vi "Measurement_input_panel.vi"(0 "OK":T4, 2 "setup":T5, 5 "Setup filename":string) -> (11 "Setup filename out":string, 12 "Analysis Info cluster":T8[](array[typedef])=[{"Colour"=0, "Inst type"=enum."Pitot-static tube", "Inst name"="Manometer voltage", "Symbol"="U", "Code name"="", "Extra Info"="U", "Inst Array"=enum."PWA", "Extra Titles"=[], "Extra Values"=[], "U"=0.0, "u^2"=0.0, "u^3"=0.0, "u^4"=0.0, "Skew_u"=0.0, "Kurt_u"=0.0, "Sd Error in Mean"=0.0, "% u'/U"=0.0, "X"=0.0, "Y"=0.0, "Z"=0.0, "Timescale integral to 25%"=0.0, "Sd Error in Variance"=0.0, "Calib File"=path "", "Calib Constants"=[], "Output Position"=FALSE, "Full Stats"=FALSE, "Av Sampling Rate"=0.0, "Av No of Samples"=0.0, "Total Meas Time (s)"=0.0, "ADAM Ch Name"=""}, {"Colour"=0, "Inst type"=enum."Pitot-static tube", "Inst name"="Manometer voltage", "Symbol"="U", "Code name"="", "Extra Info"="U", "Inst Array"=enum."PWA", "Extra Titles"=[], "Extra Values"=[], "U"=0.0, "u^2"=0.0, "u^3"=0.0, "u^4"=0.0, "Skew_u"=0.0, "Kurt_u"=0.0, "Sd Error in Mean"=0.0, "% u'/U"=0.0, "X"=0.0, "Y"=0.0, "Z"=0.0, "Timescale integral to 25%"=0.0, "Sd Error in Variance"=0.0, "Calib File"=path "", "Calib Constants"=[], "Output Position"=FALSE, "Full Stats"=FALSE, "Av Sampling Rate"=0.0, "Av No of Samples"=0.0, "Total Meas Time (s)"=0.0, "ADAM Ch Name"=""}, {"Colour"=0, "Inst type"=enum."Pitot-static tube", "Inst name"="Manometer voltage", "Symbol"="U", "Code name"="", "Extra Info"="U", "Inst Array"=enum."PWA", "Extra Titles"=[], "Extra Values"=[], "U"=0.0, "u^2"=0.0, "u^3"=0.0, "u^4"=0.0, "Skew_u"=0.0, "Kurt_u"=0.0, "Sd Error in Mean"=0.0, "% u'/U"=0.0, "X"=0.0, "Y"=0.0, "Z"=0.0, "Timescale integral to 25%"=0.0, "Sd Error in Variance"=0.0, "Calib File"=path "", "Calib Constants"=[], "Output Position"=FALSE, "Full Stats"=FALSE, "Av Sampling Rate"=0.0, "Av No of Samples"=0.0, "Total Meas Time (s)"=0.0, "ADAM Ch Name"=""}] {"Sd Error in Variance" format="%.2f"; "Skew_u" format="%.2f"; "% u'/U" format="%.2f"; "Sd Error in Mean" format="%.2f"; "Kurt_u" format="%.2f"; "u^4" format="%.2f"; "u^3" format="%.2f"; "U" format="%.2f"; "u^2" format="%.2f"})   [LabVIEW 2013]
uses:
  Controls/Ch_and_spans_choices.ctl
  Controls/Inst_type.ctl
  Controls/Analysis_info_cluster.ctl
  Controls/Instrument_Array.ctl
  Controls/LDA_Setup.ctl
  Controls/Setup.ctl
  Controls/ok_button.ctl
  Controls/Trigger_Mode.ctl
  Controls/PWA_Data.ctl
  File/Setup_Filetype.ctl
  Controls/Post_Process.ctl
  Controls/App_Global.ctl
  Controls/Ch_and_Spans.ctl
  Globals/Meas_global.vi
  Globals/Trav_pos_global.vi
  Globals/LDA_meas_global_1.vi
  Globals/Preference_global.vi
panel:
  in  "Acquisition Plug in":u16(ring) items=["ADAM_Server_Channels.vi", "Channels_and_Index.ctl", "DataTranslation.vi", "DT_With_Multiplexer.vi", "LDA_IP.vi", "NI-DAQmx.vi", "Simulate_kernal.vi"]
  in  "Select Duplicate Channels":bool
  in  "PWA Data":T1
  out "Inst type":T2
  in  "Edit temp and Press":bool
  out "Abs Press (mbar)":dbl=1013.0 format="%.1f"
  out "Temp (deg C)":dbl=21.0 format="%.1f"
  in  "Trigger mode":T3
  in  "Select Plug Ins":bool
  in  "Sync Delay Time (ms)":dbl=24.0 format="%.2f"
  out "XW Present?":bool
  out "Read Setup File?":bool
  out "Setup Paths":string[](array[string])
  in  "Select ADAM Channels":bool
  in  "stop":bool
  out "Notes":string
  in  "Setup filename selector":u16(ring) items=["Current_Setup.xls", "Calib_Setup.xls"]
  in  "Synchronise Analogue channels with LDA":bool
  in  "LDA set up":T6={"dimensions"=enum."2D", "Analogue Freq Multiplier"=0.1} {"Analogue Freq Multiplier" min=0.1 max=100.0 format="%_5g"}
  in  "LDA data":enum16{"No LDA data", "Take LDA data"}(ring)=enum."Take LDA data"
  in  "Cross wire":T7(ring)
  in  "No of Analogue inst":i32=1
  in  "Ch & spans choices":T10[](array[typedef]) {"D" format="%.2f"; "Ch No" min=0; "low limit" min=-10 max=10 format="%.2f"; "high limit" min=-10 max=10 format="%.2f"}
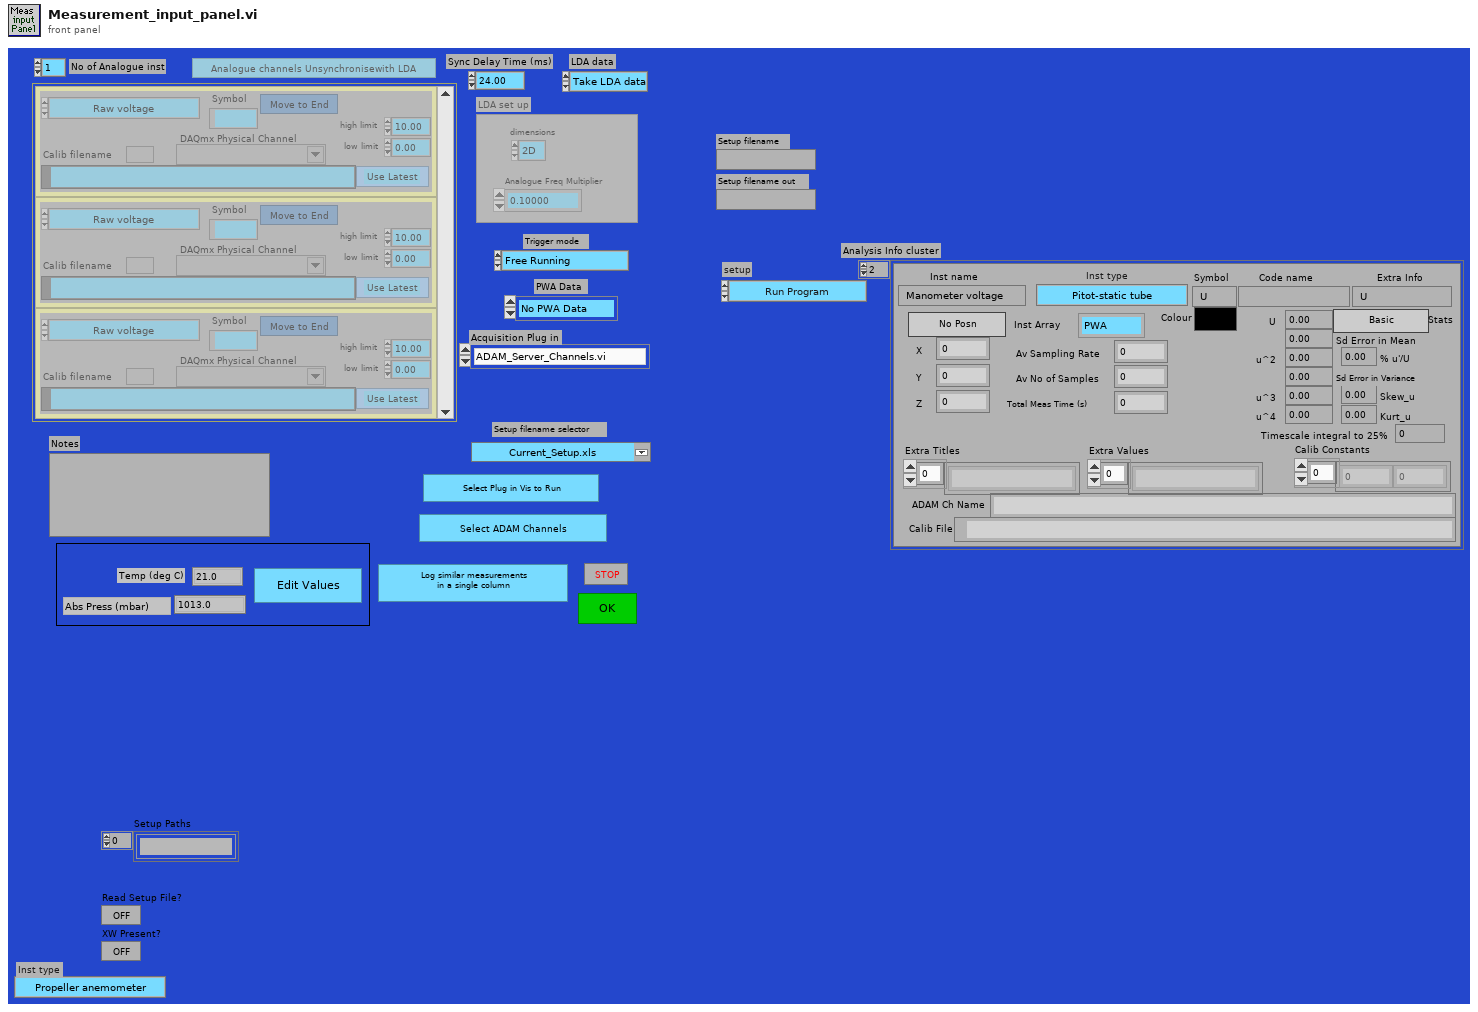
[diagram p1: front panel]
types:
  T1 = typedef "PWA_Data.ctl" = enum16{"No PWA Data", "One Ch PWA"}
  T2 = typedef "Inst_type.ctl" = enum16{"Propeller anemometer", "Raw voltage", "Pressure Transducer", "Pitot-static tube", "Preston tube", "Hot wire", "Cross wire 1", "Cross wire 2", "Generic Linear", "Generic Polynomial", "Generic BackPoly", "Fast FID", "Thermocouple", "Cold wire", "Pulsed Wire", "LDA Vel", "LDA Tran time", "LDA Arr time"}
  T3 = typedef "Trigger_Mode.ctl" = enum16{"Free Running", "Start on Trigger", "Trigger Every Block", "Trigger Every Sample"}
  T4 = typedef "ok_button.ctl" = bool
  T5 = typedef "Setup.ctl" = enum16{"Run Program", "Show Setup", "Save Current Setup", "Setup Front Panel"}
  T6 = typedef "LDA_Setup.ctl" = cluster{"dimensions":enum16{"1D", "2D"}, "Analogue Freq Multiplier":dbl}
  T7 = enum16{"2nd component as calculated", "2nd component multipled by -1"}
  T8 = typedef "Analysis_info_cluster.ctl" = cluster{"Colour":u32, "Inst type":T2, "Inst name":string, "Symbol":string, "Code name":string, "Extra Info":string, "Inst Array":T9, "Extra Titles":string[], "Extra Values":string[], "U":dbl, "u^2":dbl, "u^3":dbl, "u^4":dbl, "Skew_u":dbl, "Kurt_u":dbl, "Sd Error in Mean":dbl, "% u'/U":dbl, "X":dbl, "Y":dbl, "Z":dbl, "Timescale integral to 25%":dbl, "Sd Error in Variance":dbl, "Calib File":path, "Calib Constants":dbl[], "Output Position":bool, "Full Stats":bool, "Av Sampling Rate":dbl, "Av No of Samples":dbl, "Total Meas Time (s)":dbl, "ADAM Ch Name":string}
  T9 = typedef "Instrument_Array.ctl" = enum16{"PWA", "LDA", "Analogue"}
  T10 = typedef "Ch_and_spans_choices.ctl" = cluster{"high limit":sgl, "low limit":sgl, "Ch No":i16, "Calib filename":path, "Inst type":T2, "Symbol":string, "Move channel":bool, "Use Latest":bool, "D":dbl, "Ch Name":string, "DAQmx Physical Channel":tag}
  T11 = typedef "Post_Process.ctl" = enum16{"Take New Data", "Post Process Raw Data File"}
  T12 = typedef "Setup_Filetype.ctl" = enum16{"Measurement Setups", "Calibration Setups", "General", "Results File Plotter Setups", "Speed Calib Tweaks"}
  T13 = typedef "App_Global.ctl" = enum16{"Read Global", "Write to Global", "Initialise Array"}
  T14 = typedef "Ch_and_Spans.ctl" = cluster{"high limit (10V)":sgl, "low limit (-10V)":sgl, "Ch No":i16, "Var name":string, "Use Latest Calib":bool, "DAQmx Chan":tag}
  T15 = enum16{"Zero or one", "One", "Zero or more", "One or more"}
  T16 = typedef "Traverse_cluster.ctl" = cluster{"Start X":dbl, "Start Y":dbl, "Start Z":dbl, "End X":dbl, "End Y":dbl, "End Z":dbl, "No. of pts.":i32, "Spacing":T17, "Filename":path, "Tunnel Speed":dbl, "Averaging time (min)":dbl, "Extra Commands":string, "Specific Arguments":string, "Emission Rate (l/min)":dbl, "Trace Gas Concentration (%)":dbl, "Density Ratio":string, "Comments":string, "Row No":i32, "Row Type Selector":T18, "Completion time":string, "Row Duration (mins)":dbl, "No. of Valid pts.":i32, "Meas Setup File":string}
  T17 = typedef "Spacing.ctl" = enum16{"Linear", "Log", "Gauss", "Specified", "N/A"}
  T18 = typedef "Multi_run_mode.ctl" = enum16{"Move Traverse Only", "Set Tunnel Speed Only", "Set Source Only", "Set Measurement Conditions", "Single Measurement", "Vertical Profile", "Lateral Profile", "Longitudinal Profile", "Explore Volume", "Multi-Axis Profile", "Auto Calibrate", "Meas Fast FID Bkgnd", "Check Beam Power", "Scanning Valve Measurement", "Run VI Named:", "Set ADAM Ch", "Wait (minutes)", "Send Message", "Synchronize With:", "Fall Back to this Row", "Turn Off Row Repeating", "Blank Row", "Traverse 3D Volume"}
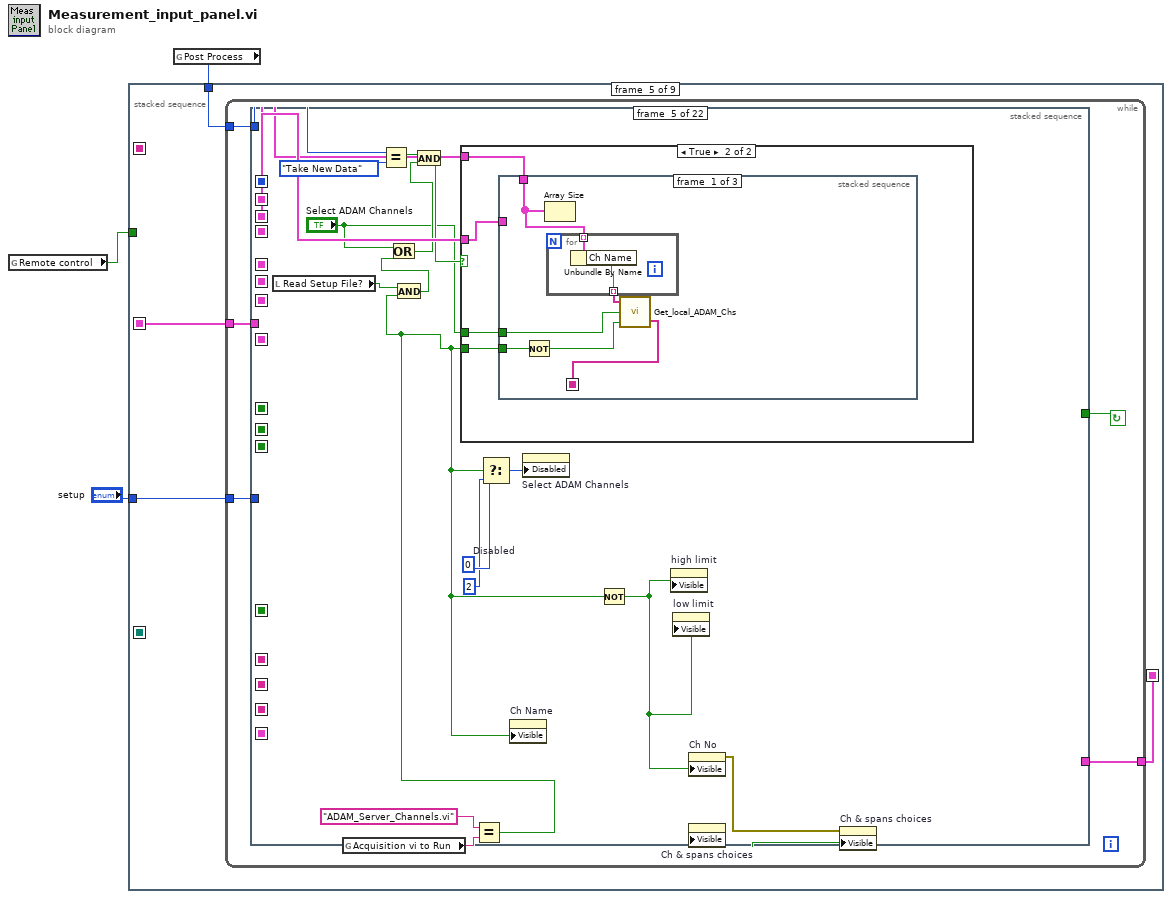
[diagram p0: block diagram]
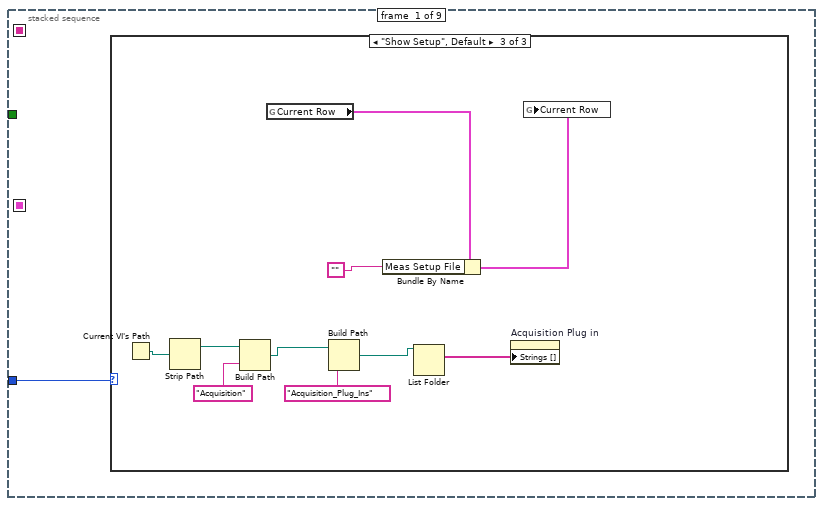
[diagram p2: hidden frame]
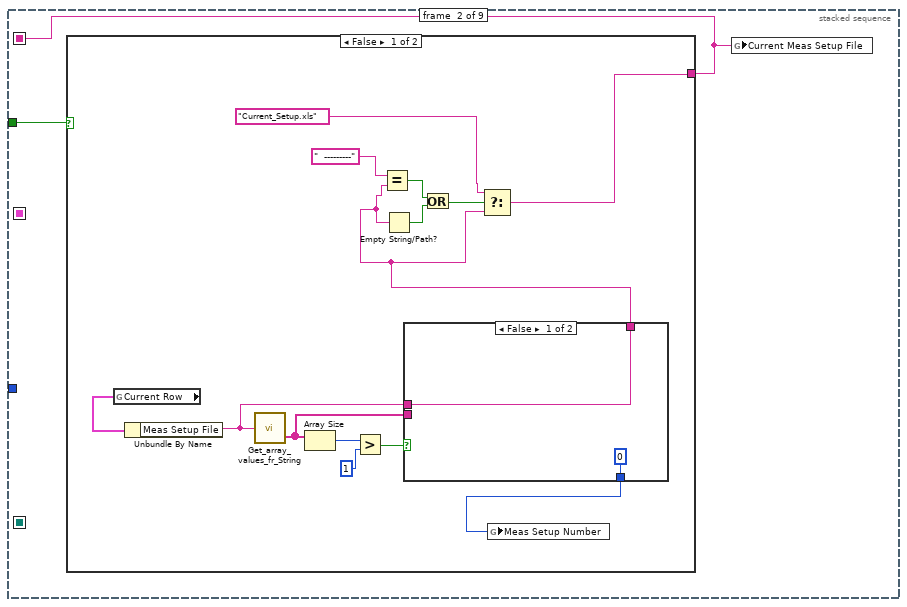
[diagram p5: hidden frame]
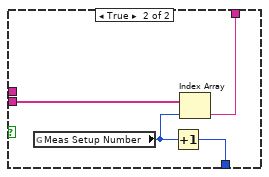
[diagram p6: hidden frame]
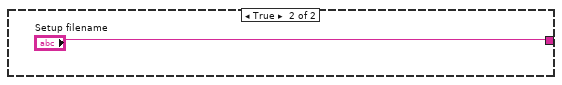
[diagram p7: hidden frame]
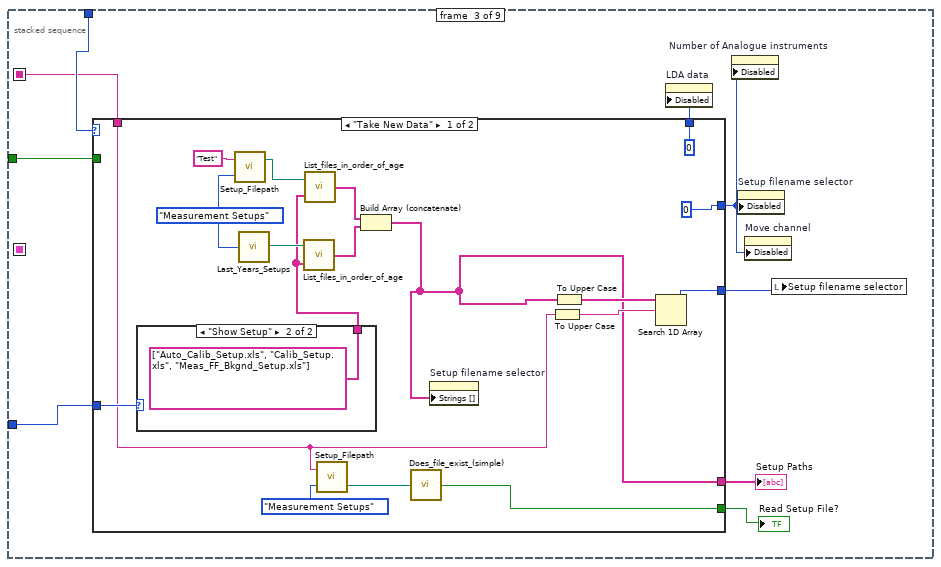
[diagram p8: hidden frame]
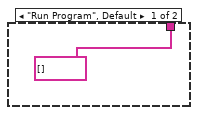
[diagram p9: hidden frame]
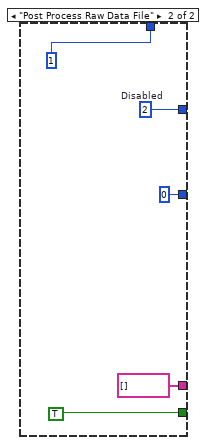
[diagram p10: hidden frame]
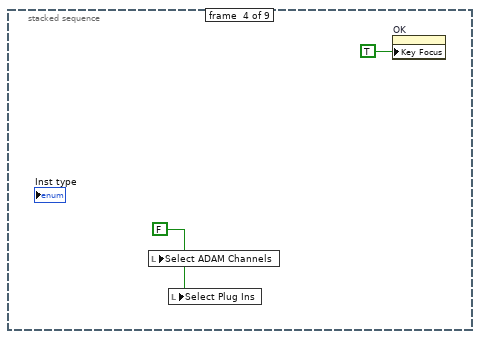
[diagram p11: hidden frame]
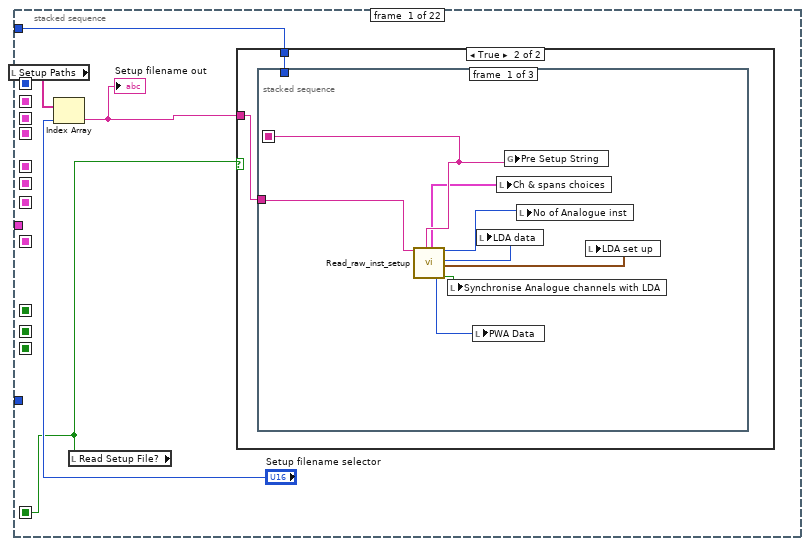
[diagram p12: hidden frame]
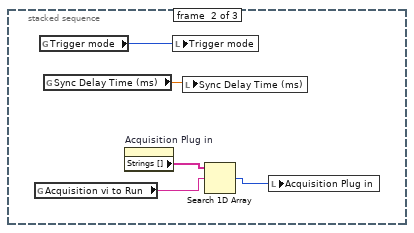
[diagram p14: hidden frame]
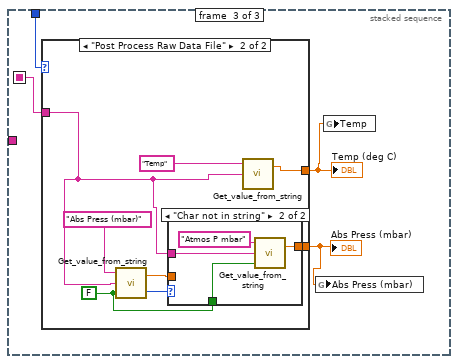
[diagram p15: hidden frame]
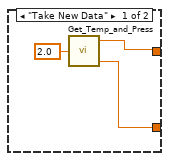
[diagram p16: hidden frame]
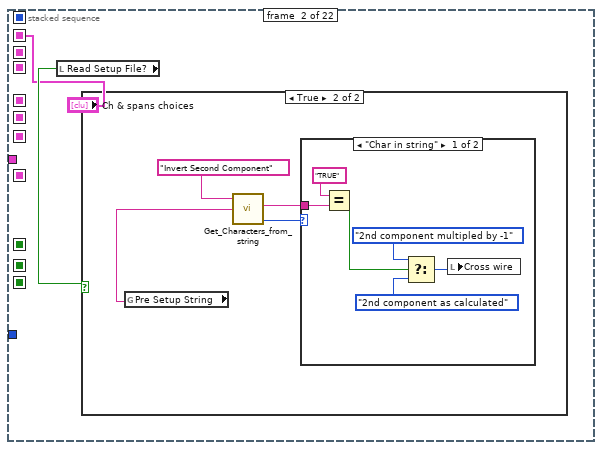
[diagram p18: hidden frame]
diagram:
  n1 = global read "Meas_global.vi" "Remote control"() -> (w1:bool)
  n2 = global read "Meas_global.vi" "Post Process"() -> (w3:T11)
  n3 = stacked-sequence {
    seq-local: [_ _ _ _ w77 _ _ _ _] -> [_ _ _ _ _ _ w748 w849 _]
    seq-local: [_ w15 _ _ _ _ _ _ _] -> [_ _ w38 _ _ _ w747 _ _]
    seq-local: [_ _ _ _ w74 _ _ _ _] -> [_ _ _ _ _ _ _ _ w912]
    seq-local: [_ _ _ _ _ _ _ w848 _] -> [_ _ _ _ _ _ _ _ w911]
    tunnel: w3 -> [_ _ w46 _ w76 _ _ w850 _]
    tunnel: "setup" -> [w4 _ w40 _ w75 _ w749 _ _]
    tunnel: w1 -> [_ w16 w39 _ _ _ _ _ _]
    frame #0 {
      n4 = case shown="\"Show Setup\", Default" w4 {
        frame "Run Program" {
        }
        frame "Setup Front Panel" {
        }
        frame "Show Setup", Default {
          n5 = Current VI's Path() -> (path=w11:path)
          n6 = Strip Path(path=w11) -> (stripped path=w10:path)  [unwired: 1 out]
          n7 = Build Path(base path=w10, name or relative path="Acquisition") -> (appended path=w7:path)
          n8 = global read "Trav_pos_global.vi" "Current Row"() -> (w14:T16)
          n9 = Build Path(base path=w7, name or relative path="Acquisition_Plug_Ins") -> (appended path=w6:path)
          n10 = Bundle By Name(cluster=w14, "Meas Setup File"="") -> (w13:T16)
          n11 = List Folder(path=w6) -> (filenames=w5:string[])  [unwired: 3 in, 3 out]
          n12 = property on="Acquisition Plug in" class="Ring (strict)"("Strings []"=w5) -> ()  [unwired: 2 in, 2 out]
          n13 = global write "Trav_pos_global.vi" "Current Row"(w13) -> ()
        }
      }
    }
    frame #1 {
      n14 = case shown="False" w16 {
        tunnel: [w29 "Setup filename"] -> w15
        frame False {
          n15 = global read "Trav_pos_global.vi" "Current Row"() -> (w25:T16)
          n16 = Unbundle By Name(w25) -> ("Meas Setup File"=w19:string)
          n17 = call "Get_array_values_fr_String.vi"("String Value"=w19) -> ("String array"=w18:string[])  [unwired: 1 out]
          n18 = Array Size(array=w18) -> (size(s)=w23:i32)
          n19 = Greater?(x=w23, y=1) -> (0:w21:bool)
          n20 = case shown="False" w21 {
            tunnel: [w32 w35] -> w20
            tunnel: w19 -> [w32 _]
            tunnel: w18 -> [_ w36]
            tunnel: [0 w33] -> w17
            frame False {
            }
            frame True {
              n21 = global read "Trav_pos_global.vi" "Meas Setup Number"() -> (w34:i32)
              n22 = Increment(x=w34) -> (x+1=w33:i32)
              n23 = Index Array(array=w36, index=w34) -> (element=w35:string)
            }
          }
          n24 = Equal?(x="  ---------" ("f"), y=w20) -> (x = y?=w28:bool)
          n25 = Empty String/Path?(string/path=w20) -> (empty?=w27:bool)
          n26 = Or(x=w28, y=w27) -> (x .or. y?=w24:bool)
          n27 = Select(t="Current_Setup.xls", s=w24, f=w20) -> (s? t:f=w29:string)
          n28 = global write "Trav_pos_global.vi" "Meas Setup Number"(w17) -> ()
        }
        frame True {
        }
      }
      n29 = global write "Trav_pos_global.vi" "Current Meas Setup File"(w15) -> ()
    }
    frame #2 {
      n30 = case shown="\"Take New Data\"" w46 {
        tunnel: [w47 string[] []] -> w42
        tunnel: [w60 TRUE ("exists")] -> w41
        tunnel: [u8 0 ("Disabled") w68] -> w43
        tunnel: [u8 0 ("Disabled") u8 1 ("Disabled")] -> w45
        tunnel: w38 -> [w56 _]
        tunnel: [w63 0 ("index of element")] -> w44
        tunnel: w40 -> [w58 _]
        tunnel: w39 -> [_ _]
        frame "Take New Data" {
          w50 = Setup_Filetype."Measurement Setups" ("Setup File Type")
          n31 = case shown="\"Show Setup\"" w58 {
            tunnel: [string[] [] ("file names") string[] ["Auto_Calib_Setup.xls", "Calib_Setup.xls", "Meas_FF_Bkgnd_Setup.xls"] ("file names")] -> w48
            frame "Run Program", Default {
            }
            frame "Show Setup" {
            }
          }
          n32 = call "Setup_Filepath.vi"("Setup File Type"=w50, "Filename in"="Test") -> ("Directory"=w51:path)  [unwired: 1 out]
          n33 = call "Last_Years_Setups.vi"("Setup File Type"=w50) -> ("Directory"=w49:path)
          n34 = call "List_files_in_order_of_age.vi"("Files to Hide"=w48, "Folder"=w49) -> ("file names"=w53:string[])
          n35 = call "List_files_in_order_of_age.vi"("Files to Hide"=w48, "Folder"=w51) -> ("file names"=w52:string[])
          n36 = call "Setup_Filepath.vi"("Setup File Type"=Setup_Filetype."Measurement Setups", "Filename in"=w56) -> ("Filename Out"=w55:path)  [unwired: 1 out]
          n37 = Build Array (concatenate)(w52, w53) -> (w47:string[])
          n38 = call "Does_file_exist_(simple).vi"("Pathname"=w55) -> ("exists?"=w60:bool)
          n39 = property on="Setup filename selector" class="Ring (strict)"("Strings []"=w47) -> ()  [unwired: 2 in, 2 out]
          n40 = To Upper Case(1:w56) -> (0:w61:string)
          n41 = To Upper Case(1:w47) -> (0:w62:string[])
          n42 = Search 1D Array(1D array=w62, element=w61) -> (index of element=w63:i32)  [unwired: 1 out]
        }
        frame "Post Process Raw Data File" {
          w68 = u8 2  # Disabled
        }
      }
      "Setup Paths" <- w42
      "Read Setup File?" <- w41
      n43 = property on="LDA data" class="Enum (strict)"("Disabled"=w45) -> ()  [unwired: 2 in, 2 out]
      n44 = property on="Number of Analogue instruments" class="DigNum (strict)"("Disabled"=w43) -> ()  [unwired: 2 in, 2 out]
      n45 = property on="Setup filename selector" class="Ring (strict)"("Disabled"=w43) -> ()  [unwired: 2 in, 2 out]
      n46 = property on="Move channel" class="Bool (strict)"("Disabled"=w43) -> ()  [unwired: 2 in, 2 out]
      n47 = local write "Setup filename selector"(w44) -> ()
    }
    frame #3 {
      w73 = FALSE ("Select Local ADAM Channels")
      n48 = local write "Select ADAM Channels"(w73) -> ()
      n49 = local write "Select Plug Ins"(w73) -> ()
      n50 = property on="OK" class="Bool"("Key Focus"=TRUE) -> ()  [unwired: 2 in, 2 out]
    }
    frame #4 {
      n51 = while {
        tunnel: w75 -> [w79]
        tunnel: w76 -> [w80]
        tunnel: [w82] -> w77
        tunnel: [w78] -> w74
        stop <- w81 continue-if-true
        n52 = stacked-sequence {
          seq-local: [_ _ _ _ _ _ _ _ _ w243 _ _ _ _ _ _ _ _ _ _ _ _] -> [_ _ _ _ _ _ _ _ _ _ _ w306 w351 w422 _ _ _ _ _ _ _ _]
          seq-local: [_ _ _ _ w166 _ _ _ _ _ _ _ _ _ _ _ _ _ _ _ _ _] -> [_ _ _ _ _ _ w205 _ w239 w244 _ _ _ _ _ _ _ _ _ _ _ _]
          seq-local: [_ _ _ _ _ _ w210 _ _ _ _ _ _ _ _ _ _ _ _ _ _ _] -> [_ _ _ _ _ _ _ _ _ w245 _ _ _ _ _ _ _ _ _ _ _ _]
          seq-local: [_ _ _ _ _ _ _ _ _ _ _ w308 _ _ _ _ _ _ _ _ _ _] -> [_ _ _ _ _ _ _ _ _ _ _ _ w353 _ _ _ _ _ _ _ _ w713]
          seq-local: [_ _ _ _ _ _ _ _ _ _ _ _ _ _ w470 _ _ _ _ _ _ _] -> [_ _ _ _ _ _ _ _ _ _ _ _ _ _ _ w495 _ _ _ _ _ _]
          seq-local: [_ _ _ _ _ _ _ _ _ _ _ _ _ _ _ w491 _ _ _ _ _ _] -> [_ _ _ _ _ _ _ _ _ _ _ _ _ _ _ _ w519 w586 _ _ w689 w714]
          seq-local: [_ _ _ _ _ _ _ _ _ _ _ _ w357 _ _ _ _ _ _ _ _ _] -> [_ _ _ _ _ _ _ _ _ _ _ _ _ _ w467 _ _ _ _ _ _ _]
          seq-local: [_ _ _ _ _ _ _ _ _ _ _ _ _ w423 _ _ _ _ _ _ _ _] -> [_ _ _ _ _ _ _ _ _ _ _ _ _ _ w466 _ _ _ _ _ _ _]
          seq-local: [_ _ _ _ _ _ _ _ _ _ w303 _ _ _ _ _ _ _ _ _ _ _] -> [_ _ _ _ _ _ _ _ _ _ _ w307 w354 _ _ _ _ _ _ _ _ w712]
          seq-local: [_ _ _ _ _ _ _ _ _ _ _ _ _ _ _ _ w518 _ _ _ _ _] -> [_ _ _ _ _ _ _ _ _ _ _ _ _ _ _ _ _ w589 _ _ _ _]
          seq-local: [_ _ _ _ _ _ _ _ _ _ _ _ _ _ _ _ w517 _ _ _ _ _] -> [_ _ _ _ _ _ _ _ _ _ _ _ _ _ _ _ _ w588 _ _ _ _]
          seq-local: [_ _ _ _ _ _ _ _ _ _ _ _ _ _ _ _ w516 _ _ _ _ _] -> [_ _ _ _ _ _ _ _ _ _ _ _ _ _ _ _ _ w587 _ _ _ _]
          seq-local: [_ _ _ _ _ _ _ _ _ _ _ _ _ _ _ _ _ w585 _ _ _ _] -> [_ _ _ _ _ _ _ _ _ _ _ _ _ _ _ _ _ _ _ w639 _ _]
          seq-local: [_ "Ch & spans choices" _ _ _ _ _ _ _ _ _ _ _ _ _ _ _ _ _ _ _ _] -> [_ _ _ _ w157 _ _ _ _ _ _ _ _ _ _ _ _ _ w634 _ _ _]
          seq-local: [_ _ _ _ _ _ _ _ _ _ _ _ _ _ _ _ _ w583 _ _ _ _] -> [_ _ _ _ _ _ _ _ _ _ _ _ _ _ _ _ _ _ w633 _ _ _]
          seq-local: [w83 _ _ _ _ _ _ _ _ _ _ _ _ _ _ _ _ _ _ _ _ _] -> [_ _ _ _ _ _ _ _ _ _ _ _ _ _ _ _ _ w582 _ _ _ _]
          tunnel: [_ _ _ _ _ _ _ _ _ _ _ _ _ _ _ w491 _ _ _ _ _ _] -> w82
          tunnel: [_ _ _ _ _ _ _ _ _ _ _ _ w355 _ _ _ _ _ _ _ _ _] -> w81
          tunnel: w80 -> [w85 _ _ w139 w163 _ _ _ _ _ w304 _ w352 _ w469 _ _ _ _ _ w690 _]
          tunnel: w79 -> [_ _ w135 _ _ w191 _ _ _ _ _ _ _ _ w468 _ _ _ _ w641 _ _]
          tunnel: [_ _ _ _ _ _ _ _ _ _ _ _ _ _ _ _ _ w585 _ _ _ _] -> w78
          frame #0 {
            n53 = local read "Setup Paths"() -> (w87:string[])
            n54 = Index Array(array=w87, index="Setup filename selector") -> (element=w84:string)
            "Setup filename out" <- w84
            n55 = local read "Read Setup File?"() -> (w83:bool)
            n56 = case shown="True" w83 {
              tunnel: w84 -> [_ w89]
              tunnel: w85 -> [_ w88]
              frame False {
              }
              frame True {
                n57 = stacked-sequence {
                  seq-local: [w92 _ _] -> [_ _ w105]
                  tunnel: w89 -> [w94 _ _]
                  tunnel: w88 -> [_ _ w106]
                  frame #0 {
                    n58 = call "Read_raw_inst_setup.vi"("Setup file"=w94) -> ("Setup string"=w92:string, "Ch & spans choices"=w90:T10[], "PWA Data"=w91:T1, "Number of Analogue instruments"=w97:i32, "LDA data"=w96:enum16{"No LDA data", "Take LDA data"}, "LDA set up"=w93:T6, "Synchronise Analogue channels with LDA"=w95:bool)  [unwired: 12 out]
                    n59 = local write "Synchronise Analogue channels with LDA"(w95) -> ()
                    n60 = local write "PWA Data"(w91) -> ()
                    n61 = local write "LDA data"(w96) -> ()
                    n62 = local write "Ch & spans choices"(w90) -> ()
                    n63 = global write "Meas_global.vi" "Pre Setup String"(w92) -> ()
                    n64 = local write "No of Analogue inst"(w97) -> ()
                    n65 = local write "LDA set up"(w93) -> ()
                  }
                  frame #1 {
                    n66 = global read "Meas_global.vi" "Acquisition vi to Run"() -> (w99:string)
                    n67 = global read "Meas_global.vi" "Trigger mode"() -> (w101:T3)
                    n68 = global read "LDA_meas_global_1.vi" "Sync Delay Time (ms)"() -> (w102:dbl)
                    n69 = property on="Acquisition Plug in" class="Ring (strict)"() -> ("Strings []"=w100:string[])  [unwired: 2 in, 2 out]
                    n70 = local write "Trigger mode"(w101) -> ()
                    n71 = local write "Sync Delay Time (ms)"(w102) -> ()
                    n72 = Search 1D Array(1D array=w100, element=w99) -> (index of element=w98:i32)  [unwired: 1 in]
                    n73 = local write "Acquisition Plug in"(w98) -> ()
                  }
                  frame #2 {
                    n74 = case shown="\"Post Process Raw Data File\"" w106 {
                      tunnel: w105 -> [_ w112]
                      tunnel: [w107 w111] -> w103
                      tunnel: [w108 w110] -> w104
                      frame "Take New Data" {
                        n75 = call "Get_Temp_and_Press.vi"("Averaging time (mins)"=2.0) -> ("Abs Press (mbar)"=w107:dbl, "Temperature"=w108:dbl)  [unwired: 3 out]
                      }
                      frame "Post Process Raw Data File" {
                        w114 = FALSE ("Show Dialog?")
                        n76 = call "Get_value_from_string.vi"("Show Dialog?"=w114, "Input string"=w112, "Variable name"="Abs Press (mbar)") -> ("Status"=w116:enum16{"Char in string", "Char not in string"}, "Value"=w115:dbl)
                        n77 = case shown="\"Char not in string\"" w116 {
                          tunnel: [w118 w121] -> w111
                          tunnel: w115 -> [w118 _]
                          tunnel: w114 -> [_ w120]
                          tunnel: w112 -> [_ w119]
                          frame "Char in string" {
                          }
                          frame "Char not in string" {
                            n78 = call "Get_value_from_string.vi"("Show Dialog?"=w120, "Input string"=w119, "Variable name"="Atmos P mbar") -> ("Value"=w121:dbl)  [unwired: 1 out]
                          }
                        }
                        n79 = call "Get_value_from_string.vi"("Input string"=w112, "Variable name"="Temp") -> ("Value"=w110:dbl)  [unwired: 1 in, 1 out]
                      }
                    }
                    "Abs Press (mbar)" <- w103
                    "Temp (deg C)" <- w104
                    n80 = global write "Meas_global.vi" "Abs Press (mbar)"(w103) -> ()
                    n81 = global write "Meas_global.vi" "Temp"(w104) -> ()
                  }
                }
              }
            }
          }
          frame #1 {
            n82 = local read "Read Setup File?"() -> (w124:bool)
            n83 = case shown="True" w124 {
              frame False {
              }
              frame True {
                n84 = global read "Meas_global.vi" "Pre Setup String"() -> (w127:string)
                n85 = call "Get_Characters_from_string.vi"("Input string"=w127, "Variable name"="Invert Second Component") -> ("Status"=w126:enum16{"Char in string", "Char not in string"}, "Value"=w125:string)  [unwired: 1 in]
                n86 = case shown="\"Char in string\"" w126 {
                  tunnel: w125 -> [w134 _]
                  frame "Char in string" {
                    n87 = Equal?(x="TRUE", y=w134) -> (x = y?=w130:bool)
                    n88 = Select(t=T7."2nd component multipled by -1" ("Cross wire/LDA"), s=w130, f=T7."2nd component as calculated" ("Cross wire/LDA")) -> (s? t:f=w132:T7)
                    n89 = local write "Cross wire"(w132) -> ()
                  }
                  frame "Char not in string" {
                  }
                }
              }
            }
          }
          frame #2 {
            n90 = case shown="\"Show Setup\"" w135 {
              frame "Run Program", Default {
              }
              frame "Show Setup" {
                n91 = property on="Acquisition Plug in" class="Ring (strict)"() -> ("Strings []"=w138:string[])  [unwired: 2 in, 2 out]
                n92 = Index Array(array=w138, index="Acquisition Plug in") -> (element=w136:string)
                n93 = global write "Meas_global.vi" "Acquisition vi to Run"(w136) -> ()
              }
            }
          }
          frame #3 {
            n94 = case shown="True" "Edit temp and Press" {
              tunnel: w139 -> [_ w141]
              frame False {
              }
              frame True {
                n95 = case shown="\"Take New Data\"" w141 {
                  frame "Take New Data" {
                    n96 = stacked-sequence {
                      frame #0 {
                        w142 = TRUE  # Wait until done
                        n97 = call "Run_Enter_Temp.vi"("Wait until done"=w142) -> ()  [unwired: 1 out]
                      }
                      frame #1 {
                        n98 = call "Get_Temp_and_Press.vi"("Averaging time (mins)"=2.0) -> ("Abs Press (mbar)"=w143:dbl, "Temperature"=w144:dbl)  [unwired: 3 out]
                        n99 = local write "Temp (deg C)"(w144) -> ()
                        n100 = local write "Abs Press (mbar)"(w143) -> ()
                      }
                    }
                  }
                  frame "Post Process Raw Data File" {
                  }
                }
              }
            }
          }
          frame #4 {
            w159 = u8 0  # Disabled
            n101 = local read "Read Setup File?"() -> (w156:bool)
            n102 = global read "Meas_global.vi" "Acquisition vi to Run"() -> (w155:string)
            n103 = Equal?(x=w163, y=Post_Process."Take New Data" ("Post Process")) -> (x = y?=w162:bool)
            n104 = Equal?(x="ADAM_Server_Channels.vi", y=w155) -> (x = y?=w153:bool)
            n105 = And(x=w156, y=w153) -> (x .and. y?=w165:bool)
            n106 = Or(x="Select ADAM Channels", y=w165) -> (x .or. y?=w160:bool)
            n107 = And(x=w162, y=w160) -> (x .and. y?=w161:bool)
            n108 = case shown="True" w161 {
              tunnel: [w167 w168] -> w166
              tunnel: w157 -> [w167 w171]
              tunnel: "Select ADAM Channels" -> [_ w170]
              tunnel: w153 -> [_ w169]
              frame False {
              }
              frame True {
                n109 = stacked-sequence {
                  seq-local: [w174 _ _] -> [_ w183 _]
                  tunnel: w171 -> [w176 w182 _]
                  tunnel: [_ w180 _] -> w168
                  tunnel: w170 -> [w177 _ w189]
                  tunnel: w169 -> [w173 _ _]
                  frame #0 {
                    n110 = Not(x=w173) -> (.not. x?=w172:bool)
                    n111 = Array Size(array=w176) -> ()  [unwired: 1 out]
                    n112 = for {
                      tunnel: w176 -> [w179] mode=indexing
                      tunnel: [w178] -> w175 mode=indexing
                      n113 = Unbundle By Name(w179) -> ("Ch Name"=w178:string)
                    }
                    n114 = call "Get_local_ADAM_Chs.vi"("Local ADAM?"=w172, "Show setup"=w177, "Desired Local ADAM Channels"=w175) -> ("Choosen Channels"=w174:string[])  [unwired: 1 out]
                  }
                  frame #1 {
                    n115 = for {
                      tunnel: [w188] -> w180 mode=indexing
                      tunnel: w183 -> [w186]
                      tunnel: w182 -> [w187] mode=indexing
                      i -> [w184]
                      n116 = Index Array(array=w186, index=w184) -> (element=w185:string)
                      n117 = Bundle By Name(cluster=w187, "Ch No"=w184, "Ch Name"=w185) -> (w188:T10)
                    }
                    n118 = Array Size(array=w180) -> (size(s)=w181:i32)
                    n119 = local write "No of Analogue inst"(w181) -> ()
                  }
                  frame #2 {
                    n120 = case shown="True" w189 {
                      frame False {
                      }
                      frame True {
                        n121 = local write "Select ADAM Channels"(FALSE ("Select Local ADAM Channels")) -> ()
                      }
                    }
                  }
                }
              }
            }
            n122 = Select(t=w159, s=w153, f=u8 2 ("Disabled")) -> (s? t:f=w150:u8)
            n123 = Equal?(x=w155, y="NI-DAQmx.vi") -> (x = y?=w147:bool)
            n124 = property on="Ch Name" class="Str"("Visible"=w153) -> ()  [unwired: 2 in, 2 out]
            n125 = property on="Select ADAM Channels" class="Bool (strict)"("Disabled"=w150) -> ()  [unwired: 2 in, 2 out]
            n126 = Not(x=w153) -> (.not. x?=w152:bool)
            n127 = property on="high limit" class="DigNum (strict)"("Visible"=w152) -> ()  [unwired: 2 in, 2 out]
            n128 = property on="low limit" class="DigNum (strict)"("Visible"=w152) -> ()  [unwired: 2 in, 2 out]
            n129 = property on="Ch No" class="DigNum (strict)"("Visible"=w152) -> (error out=w149:errorcluster)  [unwired: 2 in, 1 out]
            n130 = property on="Ch & spans choices" class="Arr (strict)"("Visible"=w147) -> ()  [unwired: 2 in, 2 out]
            n131 = Not(x=w147) -> (.not. x?=w148:bool)
            n132 = property on="Ch & spans choices" class="Arr (strict)"(error in=w149, "Visible"=w148) -> ()  [unwired: 1 in, 2 out]
          }
          frame #5 {
            n133 = case shown="True" "Select Plug Ins" {
              tunnel: w191 -> [_ w193]
              frame False {
              }
              frame True {
                n134 = stacked-sequence {
                  tunnel: w193 -> [w194 _]
                  frame #0 {
                    w198 = TRUE  # Show Panel?
                    n135 = global read "Meas_global.vi" "Pre Setup String"() -> (w197:string)
                    n136 = local write "Select Plug Ins"(FALSE ("Select Local ADAM Channels")) -> ()
                    n137 = call "Choose_Plug_In_to_Run.vi"("setup"=w194, "Show Panel?"=w198, "Setup String In"=w197) -> ("Setup String Out"=w196:string)  [unwired: 1 out]
                    n138 = global write "Meas_global.vi" "Pre Setup String"(w196) -> ()
                  }
                  frame #1 {
                    n139 = Current VI's Path() -> (path=w200:path)
                    n140 = call "Open_Close_Front_Panel.ph.vi"("Front Panel Window:Open"=TRUE, "VI path"=w200) -> ()  [unwired: 2 out]
                  }
                }
              }
            }
          }
          frame #6 {
            n141 = Initialize Array(0) -> (w212:i32[])  [unwired: 1 out]
            n142 = for {
              shift-right: [w219] -> w208
              shift-left: w212 -> [w220]
              tunnel: [w218] -> w206 mode=indexing
              tunnel: w205 -> [w217] mode=indexing
              tunnel: [w215] -> w204 mode=indexing
              n143 = Unbundle By Name(w217) -> ("Inst type"=w214:T2)
              n144 = case shown="\"LDA Vel\"" w214 {
                tunnel: w220 -> [w224 w228 w230 w234]
                tunnel: [w223 w227 w230 w233] -> w219
                tunnel: [FALSE TRUE FALSE FALSE] -> w218
                frame "Propeller anemometer", Default {
                  n145 = Build Array (concatenate)(w224, 1) -> (w223:i32[])
                }
                frame "Cross wire 1" {
                  n146 = Build Array (concatenate)(w228, 2) -> (w227:i32[])
                }
                frame "Cross wire 2" {
                }
                frame "LDA Vel" {
                  n147 = Build Array (concatenate)(w234, 1) -> (w233:i32[])
                }
              }
              n148 = Equal?(x=w214, y=Inst_type."Preston tube" ("Inst type")) -> (x = y?=w215:bool)
            }
            n149 = Build Array (concatenate)(w208, 1) -> (w207:i32[])
            n150 = Array Subset(array=w207, length="No of Analogue inst") -> (w211:i32[])  [unwired: 1 in]
            n151 = Add Array Elements(numeric array=w211) -> (sum=w210:i32)
            n152 = Or Array Elements(Boolean array=w206) -> (logical OR=→"XW Present?":bool)
            n153 = Or Array Elements(Boolean array=w204) -> (logical OR=w202:bool)
            n154 = property on="D" class="DigNum (strict)"("Visible"=w202) -> ()  [unwired: 2 in, 2 out]
          }
          frame #7 {
            "Notes" <- ""
          }
          frame #8 {
            n155 = Array Size(array=w239) -> (size(s)=w238:i32)
            n156 = Not Equal To 0?(x=w238) -> (x != 0?=w237:bool)
            n157 = case shown="True" w237 {
              tunnel: [enum16{"No Analogue data", "Take Analogue data"}."No Analogue data" ("Analogue data") enum16{"No Analogue data", "Take Analogue data"}."Take Analogue data" ("Analogue data")] -> w236
              frame False {
              }
              frame True {
              }
            }
            n158 = global write "Meas_global.vi" "Analogue data"(w236) -> ()
          }
          frame #9 {
            n159 = Index Array(array=w244, index=0) -> (element=w249:T10)
            n160 = Initialize Array(w249) -> (w247:T10[])  [unwired: 1 out]
            n161 = Build Array (concatenate)(w244, w249) -> (w248:T10[])
            n162 = for {
              N: w245 -> [_]
              tunnel: w248 -> [w257] mode=indexing
              shift-right: [w258] -> w243
              shift-left: w247 -> [w252]
              tunnel: Inst_type."Cross wire 2" ("Inst type") -> [w250]
              shift-right: [w256] -> _
              shift-left: _ -> [w255]
              tunnel: w248 -> [w254]
              n163 = Unbundle By Name(w257) -> ("Inst type"=w256:T2)
              n164 = Array Size(array=w252) -> (size(s)=w251:i32)
              n165 = Increment(x=w251) -> (x+1=w253:i32)
              n166 = case shown="\"Cross wire 1\"" w256 {
                tunnel: [w267 w288 w300] -> w258
                tunnel: w252 -> [w268 w290 w302]
                tunnel: w257 -> [w264 w291 w301]
                tunnel: w250 -> [w266 w295 _]
                tunnel: w255 -> [_ w294 _]
                tunnel: w254 -> [w271 _ _]
                tunnel: w253 -> [w270 _ _]
                frame "Cross wire 1" {
                  n167 = Index Array(array=w271, index=w270) -> (element=w265:T10)
                  n168 = Unbundle By Name(w265) -> ("Inst type"=w269:T2, "high limit"=w262:sgl, "low limit"=w261:sgl, "Ch No"=w260:i16, "Symbol"=w259:string)
                  n169 = Unbundle By Name(w264) -> ("Calib filename"=w263:path)
                  n170 = case shown="\"Cross wire 2\"" w269 {
                    tunnel: w268 -> [w281 w287]
                    tunnel: [w280 w286] -> w267
                    tunnel: w266 -> [w273 w282]
                    tunnel: w263 -> [w279 w285]
                    tunnel: w264 -> [w277 w283]
                    tunnel: w265 -> [_ _]
                    tunnel: w262 -> [w276 _]
                    tunnel: w261 -> [w275 _]
                    tunnel: w260 -> [w274 _]
                    tunnel: w259 -> [w272 _]
                    frame "Cross wire 2" {
                      n171 = Bundle By Name(cluster=w277, "Calib filename"=w279, "Inst type"=w273, "high limit"=w276, "low limit"=w275, "Ch No"=w274, "Symbol"=w272) -> (w278:T10)
                      n172 = Build Array (concatenate)(w281, w277, w278) -> (w280:T10[])
                    }
                    frame "Generic Linear", Default {
                      n173 = Bundle By Name(cluster=w283, "Calib filename"=w285, "Inst type"=w282) -> (w284:T10)
                      n174 = Build Array (concatenate)(w287, w283, w284) -> (w286:T10[])
                    }
                  }
                }
                frame "Cross wire 2" {
                  n175 = Decrement(x=w295) -> (x-1=w293:T2)
                  n176 = Equal?(x=w293, y=w294) -> (x = y?=w292:bool)
                  n177 = Bundle By Name(cluster=w291, "Inst type"=w293) -> (w289:T10)
                  n178 = case shown="False" w292 {
                    tunnel: w291 -> [_ _]
                    tunnel: w290 -> [w298 w299]
                    tunnel: w289 -> [w297 _]
                    tunnel: [w296 w299] -> w288
                    frame False {
                      n179 = Build Array (concatenate)(w298, w297) -> (w296:T10[])
                    }
                    frame True {
                    }
                  }
                }
                frame "Generic Linear", Default {
                  n180 = Build Array (concatenate)(w302, w301) -> (w300:T10[])
                }
              }
            }
          }
          frame #10 {
            n181 = Equal?(x=w304, y=Post_Process."Take New Data" ("Post Process")) -> (x = y?=w303:bool)
          }
          frame #11 {
            n182 = case shown="True" "OK" {
              tunnel: w306 -> [_ w323]
              tunnel: [FALSE w322] -> w308
              tunnel: w307 -> [_ w311]
              frame False {
              }
              frame True {
                n183 = for {
                  tunnel: w323 -> [w335] mode=indexing
                  tunnel: [w333] -> w317 mode=indexing
                  tunnel: [w329] -> w321 mode=indexing
                  n184 = Unbundle By Name(w335) -> ("high limit"=w338:sgl, "low limit"=w337:sgl, "Ch No"=w334:i16, "Inst type"=w332:T2, "Symbol"=w331:string)
                  n185 = Number To Decimal String(number=w332) -> (decimal integer string=w330:string)  [unwired: 1 out]
                  n186 = Concatenate Strings(w330, w331) -> (w329:string)
                  n187 = Greater Or Equal?(x=w338, y=w337) -> (x >= y?=w336:bool)
                  n188 = case shown="\"Propeller anemometer\", Default" w332 {
                    tunnel: w336 -> [w341 _ _ _]
                    tunnel: w334 -> [w340 _ _ _]
                    tunnel: [w339 TRUE TRUE TRUE] -> w333
                    frame "Propeller anemometer", Default {
                      n189 = case shown="False" w341 {
                        tunnel: w340 -> [w344 _]
                        tunnel: [FALSE TRUE] -> w339
                        frame False {
                          n190 = Number To Decimal String(number=w344) -> (decimal integer string=w343:string)  [unwired: 1 out]
                          n191 = Concatenate Strings("Error in input limits for Channel No ", w343) -> (w345:string)
                          n192 = One Button Dialog(message=w345) -> ()  [unwired: 2 out]
                        }
                        frame True {
                        }
                      }
                    }
                    frame "LDA Vel" {
                    }
                    frame "LDA Tran time" {
                    }
                    frame "LDA Arr time" {
                    }
                  }
                }
                n193 = call "Analyse_string_array.vi"("String array"=w321) -> ("Frequency"=w320:i32[])  [unwired: 2 out]
                n194 = global read "Meas_global.vi" "Remote control"() -> (w312:bool)
                n195 = Greater?(x=w320, y=1) -> (0:w318:bool[])
                n196 = Or Array Elements(Boolean array=w318) -> (logical OR=w314:bool)
                n197 = Compound Arithmetic op=AND(invert w312, w314, w311) -> (w313:bool)
                n198 = case shown="True" w313 {
                  tunnel: [TRUE FALSE] -> w316
                  frame False {
                  }
                  frame True {
                    n199 = Current VI's Path() -> (path=w326:path)
                    n200 = call "Open_Close_Front_Panel.ph.vi"("Front Panel Window:Open"=TRUE, "VI path"=w326) -> ()  [unwired: 2 out]
                    n201 = One Button Dialog(message="Non Unique symbol names") -> ()  [unwired: 2 out]
                  }
                }
                n202 = Build Array (concatenate)(w317, w316) -> (w315:bool[])
                n203 = And Array Elements(Boolean array=w315) -> (logical AND=w322:bool)
              }
            }
          }
          frame #12 {
            n204 = And(x=w354, y=w353) -> (x .and. y?=w356:bool)
            n205 = case shown="True" w356 {
              tunnel: w351 -> [_ w365]
              tunnel: [FALSE w364] -> w357
              tunnel: [w358 w363] -> w355
              tunnel: w353 -> [w359 _]
              tunnel: w352 -> [_ _]
              frame False {
                n206 = Not(x=w359) -> (.not. x?=w358:bool)
              }
              frame True {
                n207 = for {
                  shift-right: [w387] -> _
                  shift-left: i16[] [] -> [w386]
                  tunnel: w365 -> [w384] mode=indexing
                  tunnel: [w376] -> w366 mode=indexing
                  shift-right: [w383] -> _
                  shift-left: path[] [] -> [w382]
                  shift-right: [w370] -> _
                  shift-left: tag[] [] -> [w369]
                  n208 = Unbundle By Name(w384) -> ("Ch No"=w385:i16)
                  n209 = local read "Acquisition Plug in"() -> (w368:u16)
                  n210 = Unbundle By Name(w384) -> ("Inst type"=w381:T2, "Calib filename"=w378:path)
                  n211 = Search 1D Array(1D array=w386, element=w385) -> (index of element=w372:i32)  [unwired: 1 out]
                  n212 = Build Array (concatenate)(w386, w385) -> (w387:i16[])
                  n213 = Equal?(x=Inst_type."Fast FID" ("Inst type"), y=w381) -> (x = y?=w375:bool)
                  n214 = case shown="0, Default" w368 {
                    tunnel: w372 -> [w391 _]
                    tunnel: w385 -> [w390 _]
                    tunnel: [w388 w403] -> w371
                    tunnel: w384 -> [_ w405]
                    tunnel: [w389 w400] -> w370
                    tunnel: w369 -> [w389 w404]
                    frame 0, Default {
                      n215 = case shown="0, Default" w391 {
                        tunnel: w390 -> [w396 _]
                        tunnel: [w392 FALSE ("true")] -> w388
                        frame 0, Default {
                          n216 = Format Into String(format string="The Ch No %d appears more than once", w396) -> (resulting string=w394:string)  [unwired: 2 in, 1 out]
                          n217 = One Button Dialog(message=w394, button name ("OK")="Ok") -> (true=w392:bool)
                        }
                        frame -1 {
                        }
                      }
                    }
                    frame 5 {
                      # "NI-DAQmx"
                      n218 = Unbundle By Name(w405) -> ("DAQmx Physical Channel"=w401:tag)
                      n219 = Search 1D Array(1D array=w404, element=w401) -> (index of element=w399:i32)  [unwired: 1 in]
                      n220 = Format Into String(format string="The Ch %s appears more than once", w401) -> (resulting string=w402:string)  [unwired: 2 in, 1 out]
                      n221 = Build Array (concatenate)(w404, w401) -> (w400:tag[])
                      n222 = case shown="-1" w399 {
                        tunnel: [FALSE ("true") w409] -> w403
                        tunnel: w402 -> [_ w408]
                        frame -1 {
                        }
                        frame 1, Default {
                          n223 = One Button Dialog(message=w408, button name ("OK")="Ok") -> (true=w409:bool)
                        }
                      }
                    }
                  }
                  n224 = Search 1D Array(1D array=w382, element=w378) -> (index of element=w379:i32)  [unwired: 1 out]
                  n225 = Greater Or Equal To 0?(x=w379) -> (x >= 0?=w374:bool)
                  n226 = And(x=w375, y=w374) -> (x .and. y?=w373:bool)
                  n227 = case shown="True" w373 {
                    tunnel: [w411 FALSE ("true")] -> w377
                    tunnel: w378 -> [w410 _]
                    frame True {
                      n228 = Format Into String(format string="Calibration file %s is used more than once.", w410) -> (resulting string=w413:string)  [unwired: 2 in, 1 out]
                      n229 = One Button Dialog(message=w413, button name ("OK")="Ok") -> (true=w411:bool)
                    }
                    frame False {
                    }
                  }
                  n230 = Build Array (concatenate)(w382, w378) -> (w383:path[])
                  n231 = Or(x=w371, y=w377) -> (x .or. y?=w376:bool)
                }
                n232 = Or Array Elements(Boolean array=w366) -> (logical OR=w363:bool)
                n233 = Not(x=w363) -> (.not. x?=w364:bool)
              }
            }
          }
          frame #13 {
            n234 = global read "Meas_global.vi" "Acquisition vi to Run"() -> (w416:string)
            n235 = Equal?(x=w416, y="NI-DAQmx.vi") -> (x = y?=w418:bool)
            n236 = call "Current_Calib_Filenames.vi"("Mode"=App_Global."Read Global") -> ("Calib Filename Out"=w421:path[], "Channel Numbers Out"=w420:string[])  [unwired: 3 in]
            n237 = for {
              tunnel: w422 -> [w437] mode=indexing
              tunnel: w420 -> [w439]
              tunnel: w421 -> [w438]
              tunnel: [w436] -> w423 mode=indexing
              tunnel: w418 -> [w424]
              w435 = Inst_type."Cross wire 2"  # Inst type
              n238 = Unbundle By Name(w437) -> ("DAQmx Physical Channel"=w429:tag, "Inst type"=w428:T2, "Ch No"=w427:i16, "Use Latest"=w426:bool, "Inst type"=w425:T2)
              n239 = Not Equal?(x=w425, y=w435) -> (x != y?=w434:bool)
              n240 = Number To Decimal String(number=w427) -> (decimal integer string=w430:string)  [unwired: 1 in]
              n241 = Compound Arithmetic op=AND(w426, w434) -> (w433:bool)
              n242 = Not Equal?(x=Inst_type."Raw voltage" ("Inst type"), y=w428) -> (x != y?=w431:bool)
              n243 = case shown="True" w433 {
                tunnel: w439 -> [_ w452]
                tunnel: w430 -> [_ w451]
                tunnel: w438 -> [_ w449]
                tunnel: w437 -> [w440 w442]
                tunnel: [w440 w444] -> w436
                tunnel: w431 -> [_ w447]
                tunnel: w429 -> [_ w445]
                tunnel: w424 -> [_ w441]
                frame False {
                }
                frame True {
                  n244 = Search 1D Array(1D array=w452, element=w451) -> (index of element=w450:i32)  [unwired: 1 out]
                  n245 = Index Array(array=w449, index=w450) -> (element=w448:path)
                  n246 = Select(t=w448, s=w447, f=path "") -> (s? t:f=w443:path)
                  n247 = case shown="True" w441 {
                    tunnel: w442 -> [w453 w461]
                    tunnel: [w455 w458] -> w444
                    tunnel: w443 -> [w454 _]
                    tunnel: w449 -> [_ w460]
                    tunnel: w445 -> [_ w462]
                    tunnel: w452 -> [_ w459]
                    frame False {
                      n248 = Bundle By Name(cluster=w453, "Calib filename"=w454) -> (w455:T10)
                    }
                    frame True {
                      n249 = Search 1D Array(1D array=w459, element=w462) -> (index of element=w456:i32)  [unwired: 1 out]
                      n250 = Index Array(array=w460, index=w456) -> (element=w457:path)
                      n251 = Bundle By Name(cluster=w461, "Calib filename"=w457) -> (w458:T10)
                    }
                  }
                }
              }
            }
          }
          frame #14 {
            n252 = global read "Meas_global.vi" "Acquisition vi to Run"() -> (w463:string)
            n253 = Equal?(x=w463, y="NI-DAQmx.vi") -> (x = y?=w465:bool)
            n254 = case shown="True" w467 {
              tunnel: w466 -> [w471 w475]
              tunnel: [w471 w474] -> w470
              tunnel: w469 -> [_ _]
              tunnel: w468 -> [_ w473]
              tunnel: w465 -> [_ w472]
              frame False {
              }
              frame True {
                n255 = case shown="\"Run Program\", Default" w473 {
                  tunnel: w475 -> [w478 w490]
                  tunnel: [w477 w490] -> w474
                  tunnel: w472 -> [w476 _]
                  frame "Run Program", Default {
                    n256 = for {
                      tunnel: w478 -> [w487] mode=indexing
                      tunnel: [w488] -> w477 mode=indexing
                      tunnel: w476 -> [w485]
                      n257 = Unbundle By Name(w487) -> ("Calib filename"=w483:path, "Use Latest"=w482:bool, "Ch No"=w481:i16, "Inst type"=w480:T2, "DAQmx Physical Channel"=w479:tag)
                      n258 = Number To Decimal String(number=w481) -> (decimal integer string=w484:string)  [unwired: 1 in]
                      n259 = Select(t=w479, s=w485, f=w484) -> (s? t:f=w486:string)
                      n260 = call "Find_calibration_file.vi"("Inst type"=w480, "Ch No"=w486, "Use Latest Calib"=w482, "filename"=w483) -> ("filename out"=w489:path)
                      n261 = Bundle By Name(cluster=w487, "Calib filename"=w489) -> (w488:T10)
                    }
                  }
                  frame "Setup Front Panel" {
                  }
                }
              }
            }
          }
          frame #15 {
            w493 = 0 ("Index")
            n262 = Index Array(array=w495, index=w493) -> (element=w494:T10)
            n263 = Initialize Array(w494, w493) -> (w492:T10[])
            n264 = for {
              shift-right: [w503] -> w497
              shift-left: w492 -> [w502]
              shift-right: [w504] -> w498
              shift-left: w492 -> [w506]
              tunnel: w495 -> [w505] mode=indexing
              n265 = Unbundle By Name(w505) -> ("Move channel"=w507:bool)
              n266 = case shown="True" w507 {
                tunnel: w506 -> [w509 w515]
                tunnel: w505 -> [w511 w514]
                tunnel: [w510 w515] -> w504
                tunnel: [w508 w513] -> w503
                tunnel: w502 -> [w508 w512]
                frame False {
                  n267 = Build Array (concatenate)(w509, w511) -> (w510:T10[])
                }
                frame True {
                  n268 = Build Array (concatenate)(w512, w514) -> (w513:T10[])
                }
              }
            }
            n269 = Build Array (concatenate)(w498, w497) -> (w496:T10[])
            n270 = for {
              tunnel: w496 -> [w501] mode=indexing
              tunnel: [w499] -> w491 mode=indexing
              n271 = Bundle By Name(cluster=w501, "Move channel"=FALSE) -> (w499:T10)
            }
          }
          frame #16 {
            n272 = for {
              shift-right: [w525] -> _
              shift-left: string[] [] -> [w526]
              tunnel: [w528] -> w517 mode=indexing
              tunnel: [w522] -> w518 mode=indexing
              tunnel: w519 -> [w524] mode=indexing
              tunnel: [w521] -> w516 mode=indexing
              n273 = Unbundle By Name(w524) -> ("Inst type"=w527:T2)
              n274 = case shown="\"Raw voltage\"" w527 {
                tunnel: [w535 w539 w542 w546 w550 w554 w558 "XW" w565 w570 w573 w577] -> w522
                tunnel: ["U" "P" "U" "U" "tau" "U" "U" "W" "U" "C" "T" "T"] -> w529
                tunnel: w526 -> [w536 w540 w544 w548 w552 w556 w560 w562 w567 w571 w575 w579]
                tunnel: [w534 w538 w543 w547 w551 w555 w559 w562 w566 w569 w574 w578] -> w525
                frame "Propeller anemometer" {
                  w535 = "Prop"
                  n275 = Build Array (concatenate)(w536, w535) -> (w534:string[])
                }
                frame "Pressure Transducer" {
                  w539 = "Mano"
                  n276 = Build Array (concatenate)(w540, w539) -> (w538:string[])
                }
                frame "Raw voltage" {
                  w542 = "RV"
                  n277 = Build Array (concatenate)(w544, w542) -> (w543:string[])
                }
                frame "Pitot-static tube" {
                  w546 = "Pitot"
                  n278 = Build Array (concatenate)(w548, w546) -> (w547:string[])
                }
                frame "Preston tube" {
                  w550 = "Preston"
                  n279 = Build Array (concatenate)(w552, w550) -> (w551:string[])
                }
                frame "Hot wire" {
                  w554 = "HW"
                  n280 = Build Array (concatenate)(w556, w554) -> (w555:string[])
                }
                frame "Cross wire 1" {
                  w558 = "XW"
                  n281 = Build Array (concatenate)(w560, w558) -> (w559:string[])
                }
                frame "Cross wire 2" {
                }
                frame "Generic Linear", Default {
                  w565 = "Gen"
                  n282 = Build Array (concatenate)(w567, w565) -> (w566:string[])
                }
                frame "Fast FID" {
                  w570 = "FF"
                  n283 = Build Array (concatenate)(w571, w570) -> (w569:string[])
                }
                frame "Thermocouple" {
                  w573 = "T"
                  n284 = Build Array (concatenate)(w575, w573) -> (w574:string[])
                }
                frame "Cold wire" {
                  w577 = "CW"
                  n285 = Build Array (concatenate)(w579, w577) -> (w578:string[])
                }
              }
              n286 = call "Analyse_string_array.vi"("String array"=w525) -> ("Unique strings"=w533:string[], "Frequency"=w531:i32[])  [unwired: 1 out]
              n287 = Search 1D Array(1D array=w533, element=w522) -> (index of element=w532:i32)  [unwired: 1 out]
              n288 = Index Array(array=w531, index=w532) -> (element=w523:i32)
              n289 = Number To Decimal String(number=w523) -> (decimal integer string=w521:string)  [unwired: 1 out]
              n290 = Concatenate Strings(w521, w522, ":", w529) -> (w528:string)
            }
          }
          frame #17 {
            w592 = T8 {"Colour"=0, "Inst type"=enum."Pitot-static tube", "Inst name"="Manometer voltage", "Symbol"="U", "Code name"="", "Extra Info"="U", "Inst Array"=enum."PWA", "Extra Titles"=[], "Extra Values"=[], "U"=0.0, "u^2"=0.0, "u^3"=0.0, "u^4"=0.0, "Skew_u"=0.0, "Kurt_u"=0.0, "Sd Error in Mean"=0.0, "% u'/U"=0.0, "X"=0.0, "Y"=0.0, "Z"=0.0, "Timescale integral to 25%"=0.0, "Sd Error in Variance"=0.0, "Calib File"=path "", "Calib Constants"=[], "Output Position"=FALSE, "Full Stats"=FALSE, "Av Sampling Rate"=0.0, "Av No of Samples"=0.0, "Total Meas Time (s)"=0.0, "ADAM Ch Name"=""}  # Analysis info cluster
            n291 = local read "Acquisition Plug in"() -> (w581:u16)
            n292 = property on="Ch Name" class="Str"() -> ("Visible"=w593:bool)  [unwired: 2 in, 2 out]
            n293 = global read "Meas_global.vi" "Pre Setup String"() -> (w584:string)
            n294 = for {
              tunnel: [w596] -> w591 mode=indexing
              tunnel: w586 -> [w612] mode=indexing
              tunnel: w589 -> [w623] mode=indexing
              tunnel: T14 {"high limit (10V)"=10.0, "low limit (-10V)"=-10.0, "Ch No"=0, "Var name"="", "Use Latest Calib"=FALSE, "DAQmx Chan"=""} ("Ch and Spans") -> [w594]
              tunnel: [w626] -> w585 mode=indexing
              tunnel: w588 -> [w615] mode=indexing
              tunnel: w592 -> [w624]
              tunnel: w587 -> [w620] mode=indexing
              tunnel: w593 -> [w608]
              tunnel: w584 -> [w616]
              tunnel: [w611] -> w583 mode=indexing
              tunnel: w582 -> [w607]
              tunnel: w581 -> [w606]
              n295 = Unbundle By Name(w612) -> ("DAQmx Physical Channel"=w605:tag, "Use Latest"=w604:bool, "high limit"=w603:sgl, "low limit"=w602:sgl, "Ch No"=w601:i16, "Inst type"=w600:T2, "Symbol"=w599:string, "D"=w598:dbl, "Ch Name"=w597:string)
              n296 = Concatenate Strings(w615, "_ADAM_Ch_Name" ("string")) -> (w613:string)
              n297 = call "Get_Characters_from_string.vi"("Input string"=w616, "Variable name"=w613) -> ("Value"=w610:string)  [unwired: 1 in, 1 out]
              n298 = Empty String/Path?(string/path=w599) -> (empty?=w621:bool)
              n299 = Select(t=w620, s=w621, f=w599) -> (s? t:f=w619:string)
              n300 = Format Into String(format string="%s (%s)" ("Format String"), w623, w619) -> (resulting string=w617:string)  [unwired: 2 in, 1 out]
              n301 = Select(t=w597, s=w608, f=w617) -> (s? t:f=w595:string)
              n302 = case shown="\"Propeller anemometer\", Default" w600 {
                tunnel: [w629 w632] -> w625
                tunnel: w601 -> [w627 _]
                tunnel: w598 -> [_ w630]
                tunnel: w606 -> [_ _]
                tunnel: w605 -> [_ _]
                frame "Propeller anemometer", Default {
                  n303 = Format Into String(format string="Ch %d" ("Format String"), w627) -> (resulting string=w629:string)  [unwired: 2 in, 1 out]
                }
                frame "Preston tube" {
                  n304 = Format Into String(format string="D = %.2f" ("Format String"), w630) -> (resulting string=w632:string)  [unwired: 2 in, 1 out]
                }
              }
              n305 = Select(t=w610, s=w607, f=w597) -> (s? t:f=w609:string)
              n306 = Bundle By Name(cluster=w612, "Ch Name"=w609) -> (w611:T10)
              n307 = Bundle By Name(cluster=w594, "DAQmx Chan"=w605, "Use Latest Calib"=w604, "high limit (10V)"=w603, "low limit (-10V)"=w602, "Ch No"=w601, "Var name"=w595) -> (w596:T14)
              n308 = Bundle By Name(cluster=w624, "Extra Info"=w625, "Inst type"=w600, "Inst name"=w617, "Symbol"=w619, "Code name"=w615, "Inst Array"=Instrument_Array."Analogue", "ADAM Ch Name"=w609) -> (w626:T8)
            }
            n309 = global write "Meas_global.vi" "Ch & spans"(w591) -> ()
          }
          frame #18 {
            n310 = Not Equal?(x=w634, y=w633) -> (x != y?=w635:bool)
            n311 = case shown="True" w635 {
              tunnel: w633 -> [_ w636]
              frame False {
              }
              frame True {
                n312 = local write "Ch & spans choices"(w636) -> ()
              }
            }
          }
          frame #19 {
            n313 = global read "Meas_global.vi" "Duplicate channels"() -> (w638:i32[])
            n314 = case shown="True" "Select Duplicate Channels" {
              tunnel: w641 -> [_ _]
              tunnel: w639 -> [w649 w672]
              tunnel: w638 -> [w643 w665]
              tunnel: [w642 w664] -> w637
              frame False {
                n315 = for {
                  tunnel: w649 -> [w663] mode=indexing
                  tunnel: [w662] -> w650 mode=indexing
                  n316 = Unbundle By Name(w663) -> ("Inst type"=w662:T2)
                }
                n317 = for {
                  tunnel: w643 -> [w659] mode=indexing
                  tunnel: w650 -> [w661]
                  tunnel: [w660] -> w654 mode=indexing
                  tunnel: [w659] -> w651 mode=indexing
                  n318 = Index Array(array=w661, index=w659) -> (element=w660:T2)
                }
                n319 = Array Size(array=w649) -> (size(s)=w652:i32)
                n320 = Array Max & Min(array=w654) -> (max value=w655:T2, min value=w656:T2)  [unwired: 2 out]
                n321 = Array Max & Min(array=w651) -> (max index (indices)=w653:i32)  [unwired: 3 out]
                n322 = Array Size(array=w643) -> (size(s)=w648:i32)
                n323 = Equal?(x=w655, y=w656) -> (x = y?=w658:bool)
                n324 = Greater?(x=w648, y=1) -> (0:w645:bool)
                n325 = Greater?(x=w652, y=w653) -> (0:w657:bool)
                n326 = Compound Arithmetic op=AND(w645, w658, w657) -> (w644:bool)
                n327 = Select(t=w643, s=w644, f=i32[] [] ("32bit integer")) -> (s? t:f=w642:i32[])
              }
              frame True {
                n328 = for {
                  tunnel: w672 -> [w679] mode=indexing
                  shift-right: [w674] -> w668
                  shift-left: string[] [] -> [w675]
                  tunnel: w665 -> [w677]
                  tunnel: [w673] -> w667 mode=indexing
                  i -> [w678]
                  n329 = Unbundle By Name(w679) -> ("Inst name"=w673:string)
                  n330 = Search 1D Array(1D array=w677, element=w678) -> (index of element=w676:i32)  [unwired: 1 out]
                  n331 = case shown="0, Default" w676 {
                    tunnel: w675 -> [w682 w683]
                    tunnel: w673 -> [w681 _]
                    tunnel: [w680 w683] -> w674
                    frame 0, Default {
                      n332 = Build Array (concatenate)(w682, w681) -> (w680:string[])
                    }
                    frame -1 {
                    }
                  }
                }
                n333 = call "Select_Strings.vi"("Available Ch names"=w667, "Message"="Please select similar instruments whose results columns will be combined", "Selector mode"=T15."Zero or more", "Desired Ch names (in)"=w668) -> ("Ch Indicies Choosen"=w664:i32[])  [unwired: 4 out]
                n334 = local write "Select Duplicate Channels"(FALSE ("Select Local ADAM Channels")) -> ()
              }
            }
            n335 = global write "Meas_global.vi" "Duplicate channels"(w637) -> ()
          }
          frame #20 {
            n336 = local read "XW Present?"() -> (w686:bool)
            n337 = case shown="\"Take LDA data\"" "LDA data" {
              tunnel: [w695 w698] -> w688
              tunnel: w689 -> [_ w696]
              tunnel: w690 -> [_ _]
              tunnel: [w695 w697] -> w685
              frame "No LDA data" {
                w694 = FALSE  # Synchronise Analogue channels with LDA
                w695 = u8 2  # Disabled
                n338 = local write "Synchronise Analogue channels with LDA"(w694) -> ()
              }
              frame "Take LDA data" {
                n339 = stacked-sequence {
                  tunnel: [w699 _] -> w698
                  tunnel: [_ w701] -> w697
                  tunnel: w696 -> [_ w702]
                  frame #0 {
                    w699 = u8 0  # Disabled
                  }
                  frame #1 {
                    n340 = Array Size(array=w702) -> (size(s)=w703:i32)
                    n341 = Not Equal To 0?(x=w703) -> (x != 0?=w700:bool)
                    n342 = case shown="False" w700 {
                      tunnel: w700 -> [w705 _]
                      tunnel: [w704 w706] -> w701
                      frame False {
                        w704 = u8 2  # Disabled
                        n343 = local write "Synchronise Analogue channels with LDA"(w705) -> ()
                      }
                      frame True {
                        w706 = u8 0  # Disabled
                      }
                    }
                  }
                }
              }
            }
            n344 = property on="Cross wire/LDA" class="Enum (strict)"("Visible"=w686) -> ()  [unwired: 2 in, 2 out]
            n345 = case shown="True" w686 {
              tunnel: [w692 "Cross wire"] -> w684
              frame False {
                w692 = T7."2nd component as calculated"  # Cross wire/LDA
              }
              frame True {
              }
            }
            n346 = global write "Meas_global.vi" "Cross wire + or -ve"(w684) -> ()
            n347 = Wait (ms)(milliseconds to wait=u32 100) -> ()  [unwired: 1 out]
            n348 = property on="Synchronise Analogue channels with LDA" class="Bool (strict)"("Disabled"=w685) -> ()  [unwired: 2 in, 2 out]
            n349 = property on="LDA set up" class="Clust (strict)"("Disabled"=w688) -> ()  [unwired: 2 in, 2 out]
          }
          frame #21 {
            n350 = And(x=w712, y=w713) -> (x .and. y?=w711:bool)
            n351 = local read "Synchronise Analogue channels with LDA"() -> (w710:bool)
            n352 = while {
              shift-left: _ -> [w739]
              shift-right: [w740] -> w707
              tunnel: [w741] -> w709
              stop <- FALSE continue-if-true
              n353 = local read "Setup filename selector"() -> (w740:u16)
              n354 = Not Equal?(x=w740, y=w739) -> (x != y?=w741:bool)
            }
            n355 = case shown="True" w710 {
              tunnel: w714 -> [_ w725]
              tunnel: w711 -> [_ w724]
              frame False {
              }
              frame True {
                n356 = case shown="True" w724 {
                  tunnel: w725 -> [_ w728]
                  frame False {
                  }
                  frame True {
                    n357 = for {
                      tunnel: w728 -> [w737] mode=indexing
                      tunnel: [w730] -> w727 mode=indexing
                      n358 = Unbundle By Name(w737) -> ("Inst type"=w736:T2, "Symbol"=w734:string)
                      n359 = Equal?(x=w734, y="Sync") -> (x = y?=w732:bool)
                      n360 = Equal?(x=Inst_type."Raw voltage" ("Inst type"), y=w736) -> (x = y?=w731:bool)
                      n361 = And(x=w731, y=w732) -> (x .and. y?=w730:bool)
                    }
                    n362 = Or Array Elements(Boolean array=w727) -> (logical OR=w726:bool)
                    n363 = case shown="False" w726 {
                      frame False {
                        n364 = One Button Dialog(message="To Perform LDA Sync you must provide a Raw voltage channel having the symbol \"Sync\"") -> ()  [unwired: 2 out]
                      }
                      frame True {
                      }
                    }
                  }
                }
              }
            }
            n365 = case shown="True" w709 {
              tunnel: [FALSE ("exists?") w723] -> w708
              tunnel: w707 -> [_ w721]
              frame False {
              }
              frame True {
                n366 = local read "Setup Paths"() -> (w722:string[])
                n367 = Index Array(array=w722, index=w721) -> (element=w719:string)
                n368 = call "Setup_Filepath.vi"("Setup File Type"=Setup_Filetype."Measurement Setups", "Filename in"=w719) -> ("Filename Out"=w718:path)  [unwired: 1 out]
                n369 = call "Does_file_exist_(simple).vi"("Pathname"=w718) -> ("exists?"=w723:bool)
              }
            }
            n370 = local write "Read Setup File?"(w708) -> ()
            n371 = Current VI's Path() -> (path=w715:path)
            n372 = call "Close_Panel_and_Abort.vi"("Vi path"=w715, "stop"="stop") -> ()  [unwired: 1 out]
          }
        }
      }
    }
    frame #5 {
      n373 = local read "LDA data"() -> (w744:enum16{"No LDA data", "Take LDA data"})
      n374 = case shown="\"Take LDA data\"" w744 {
        tunnel: [FALSE ("Synchronise Analogue channels with LDA") "Synchronise Analogue channels with LDA"] -> w743
        frame "No LDA data" {
        }
        frame "Take LDA data" {
        }
      }
      n375 = global write "Meas_global.vi" "Synchronise with LDA"(w743) -> ()
      n376 = global write "Meas_global.vi" "LDA data"(w744) -> ()
      n377 = global write "Meas_global.vi" "LDA set up"("LDA set up") -> ()
    }
    frame #6 {
      n378 = stacked-sequence {
        seq-local: [_ w784 _ _] -> [_ _ _ w842]
        seq-local: [_ _ w810 _] -> [_ _ _ w841]
        seq-local: [w752 _ _ _] -> [_ _ _ w829]
        tunnel: w749 -> [w751 _ _ w833]
        tunnel: w748 -> [_ _ _ w832]
        tunnel: w747 -> [w750 _ _ _]
        frame #0 {
          n379 = local read "PWA Data"() -> (w753:T1)
          n380 = case shown="\"One Ch PWA\"" w753 {
            tunnel: ["" w762] -> w752
            tunnel: w751 -> [_ w761]
            tunnel: w750 -> [_ w757]
            frame "No PWA Data" {
            }
            frame "One Ch PWA" {
              n381 = Not Equal?(x="Calib_Setup.xls", y=w757) -> (x != y?=w756:bool)
              n382 = case shown="\"Setup Front Panel\"" w761 {
                tunnel: [w766 w769 w772 w775] -> w760
                tunnel: [w765 w768 w771 w774] -> w759
                tunnel: [w764 w767 w770 w773] -> w755
                tunnel: w756 -> [w764 w767 w770 _]
                frame "Show Setup" {
                  w766 = TRUE  # Show Panel?
                  w765 = T4 FALSE  # OK
                }
                frame "Run Program" {
                  w769 = FALSE  # Show Panel?
                  w768 = T4 TRUE  # OK
                }
                frame "Save Current Setup" {
                  w772 = FALSE  # Show Panel?
                  w771 = T4 TRUE  # OK
                }
                frame "Setup Front Panel" {
                  w773 = FALSE  # Check Calib file?
                  w775 = FALSE  # Show Panel?
                  w774 = T4 TRUE  # OK
                }
              }
              n383 = global read "Meas_global.vi" "Pre Setup String"() -> (w763:string)
              n384 = call "PWA_Setup_Panel.vi"("Show Panel?"=w760, "Check Calib file?"=w755, "OK"=w759, "Incoming Setup String"=w763) -> ("Outgoing Setup String"=w762:string)  [unwired: 3 out]
            }
          }
        }
        frame #1 {
          n385 = local read "LDA set up"() -> (w789:T6)
          n386 = global read "Meas_global.vi" "Duplicate channels"() -> (w788:i32[])
          n387 = Unbundle By Name(w789) -> ("dimensions"=w781:enum16{"1D", "2D"}, "Analogue Freq Multiplier"=w779:dbl)
          n388 = case shown="\"2D\"" w781 {
            tunnel: ["1D" "2D"] -> w783
            frame "1D" {
            }
            frame "2D" {
            }
          }
          n389 = for {
            shift-right: [w792] -> w786
            shift-left: "" -> [w795]
            tunnel: w788 -> [w796] mode=indexing
            n390 = Number To Decimal String(number=w796) -> (decimal integer string=w794:string)  [unwired: 1 out]
            n391 = Concatenate Strings(w795, w794, "; ") -> (w792:string)
          }
          n392 = call "Characters_to_string.vi"("Characters to write"=w783, "Label for characters"="LDA Dimensions") -> ("Output string"=w782:string)
          n393 = call "Value_to_string.vi"("Value"=w779, "Label for value"="LDA Analog Freq Multiplier") -> ("Output string"=w776:string)  [unwired: 1 in]
          n394 = call "Characters_to_string.vi"("Characters to write"=w786, "Label for characters"="Log_Similar_Measurements_in_the _same_column") -> ("Output string"=w777:string)
          n395 = Concatenate Strings(w782, w776, w777) -> (w784:string)
        }
        frame #2 {
          n396 = global write "Meas_global.vi" "Trigger mode"("Trigger mode") -> ()
          n397 = local read "Cross wire"() -> (w813:T7)
          n398 = global read "Preference_global.vi" "Rig Setup"() -> (w799:string)
          n399 = Match Pattern(string=w799, regular expression="-") -> (before substring=w798:string)  [unwired: 4 out]
          n400 = case shown="\"Free Running\"" "Trigger mode" {
            tunnel: ["Free Running" "Trigger Every Block" "Trigger Every Sample" "Start on Trigger"] -> w808
            frame "Free Running" {
            }
            frame "Trigger Every Block" {
            }
            frame "Trigger Every Sample" {
            }
            frame "Start on Trigger" {
            }
          }
          n401 = property on="PWA Data" class="Enum (strict)"() -> ("Strings []"=w804:string[])  [unwired: 2 in, 2 out]
          n402 = global write "Meas_global.vi" "PWA Data"("PWA Data") -> ()
          n403 = Equal?(x=T7."2nd component multipled by -1" ("Cross wire/LDA"), y=w813) -> (x = y?=w812:bool)
          n404 = case shown="\"EnFlo_Tunnel\"" w798 {
            tunnel: ["" w820] -> w797
            frame "False", Default {
            }
            frame "EnFlo_Tunnel" {
              n405 = call "Characters_to_string.vi"("Characters to write"="FALSE", "Label for characters"="Show_all_EnFlo_Tunnel_Columns") -> ("Output string"=w820:string)
            }
          }
          n406 = Index Array(array=w804, index="PWA Data") -> (element=w803:string)
          n407 = Select(t="TRUE", s=w812, f="FALSE") -> (s? t:f=w815:string)
          n408 = call "Characters_to_string.vi"("Characters to write"=w803, "Label for characters"="Pulsed_Wire_Data" ("Variable name")) -> ("Output string"=w802:string)
          n409 = call "Characters_to_string.vi"("Characters to write"=w815, "Label for characters"="Invert Second Component") -> ("Output string"=w811:string)
          n410 = call "Characters_to_string.vi"("Characters to write"=w808, "Label for characters"="Trigger mode") -> ("Output string"=w806:string)
          n411 = Concatenate Strings(w806, w802, w811, w797) -> (w810:string)
        }
        frame #3 {
          w834 = FALSE  # Show Panel?
          n412 = for {
            tunnel: w832 -> [w847] mode=indexing
            tunnel: [w846] -> w828 mode=indexing
            n413 = Unbundle By Name(w847) -> ("Ch Name"=w846:string)
          }
          n414 = global read "Meas_global.vi" "Pre Setup String"() -> (w835:string)
          n415 = call "Choose_Plug_In_to_Run.vi"("setup"=w833, "Show Panel?"=w834, "Setup String In"=w835) -> ("Setup String Out"=w836:string)  [unwired: 1 out]
          n416 = Array To Spreadsheet String(array=w828, 3:"%s" ("format string")) -> (spreadsheet string=w830:string)  [unwired: 1 out]
          n417 = call "Add_label_to_string.vi"("String to write"=w830, "File Label"="Local ADAM Channels") -> ("Output string"=w843:string)
          n418 = call "Date_and_Time_to_string.vi"() -> ("Date and time (spreadsheet)"=w838:string)
          n419 = global read "Meas_global.vi" "New Setup String"() -> (w837:string)
          n420 = call "Value_to_string.vi"("Value"="Sync Delay Time (ms)", "Label for value"="Sync Delay Time (ms)" ("Label for characters")) -> ("Output string"=w831:string)  [unwired: 1 in]
          n421 = Concatenate Strings(w837, w829, w836, w838, w842, w841, w843, w831) -> (w845:string)
          n422 = global write "Meas_global.vi" "New Setup String"(w845) -> ()
          n423 = global write "LDA_meas_global_1.vi" "Sync Delay Time (ms)"("Sync Delay Time (ms)") -> ()
        }
      }
    }
    frame #7 {
      n424 = case shown="\"Take New Data\"" w850 {
        tunnel: w849 -> [w860 w903]
        tunnel: [w858 w897] -> w848
        frame "Take New Data" {
          n425 = global read "Meas_global.vi" "Acquisition vi to Run"() -> (w856:string)
          n426 = Equal?(x=w856, y="NI-DAQmx.vi") -> (x = y?=w857:bool)
          n427 = for {
            tunnel: w860 -> [w862] mode=indexing
            shift-right: [w872] -> w854
            shift-left: string[] [] -> [w873]
            shift-right: [w870] -> w853
            shift-left: path[] [] -> [w871]
            tunnel: [w869] -> w858 mode=indexing
            tunnel: w857 -> [w861]
            n428 = Unbundle By Name(w862) -> ("DAQmx Physical Channel"=w867:tag, "Use Latest"=w866:bool, "Inst type"=w865:T2, "Ch No"=w864:i16, "Calib filename"=w863:path)
            n429 = case shown="\"Propeller anemometer\", Default" w865 {
              tunnel: w873 -> [w882 w896]
              tunnel: w864 -> [w881 _]
              tunnel: [w880 w896] -> w872
              tunnel: w871 -> [w879 w895]
              tunnel: w863 -> [w878 _]
              tunnel: [w877 w895] -> w870
              tunnel: w867 -> [w875 _]
              tunnel: w866 -> [w876 _]
              tunnel: w861 -> [w874 _]
              frame "Propeller anemometer", Default {
                n430 = case shown="False" w876 {
                  tunnel: w882 -> [w892 w894]
                  tunnel: w881 -> [w884 _]
                  tunnel: [w891 w894] -> w880
                  tunnel: w879 -> [w890 w893]
                  tunnel: w878 -> [w889 _]
                  tunnel: [w888 w893] -> w877
                  tunnel: w875 -> [w887 _]
                  tunnel: w874 -> [w883 _]
                  frame False {
                    n431 = Number To Decimal String(number=w884) -> (decimal integer string=w885:string)  [unwired: 1 in]
                    n432 = Select(t=w887, s=w883, f=w885) -> (s? t:f=w886:string)
                    n433 = Build Array (concatenate)(w890, w889) -> (w888:path[])
                    n434 = Build Array (concatenate)(w892, w886) -> (w891:string[])
                  }
                  frame True {
                  }
                }
              }
              frame "Raw voltage" {
              }
            }
            n435 = call "Current_Filepath.vi"("Filename in"=w863, "Data Type"="Calibrations") -> ("Filename Out"=w869:path)  [unwired: 1 out]
          }
          n436 = call "Current_Calib_Filenames.vi"("Calib Filename"=w853, "Channel Numbers"=w854, "Mode"=App_Global."Write to Global") -> ()  [unwired: 1 in, 2 out]
        }
        frame "Post Process Raw Data File" {
          n437 = for {
            tunnel: w903 -> [w909] mode=indexing
            tunnel: [w908] -> w897 mode=indexing
            n438 = Unbundle By Name(w909) -> ("Calib filename"=w908:path)
          }
          n439 = global read "Meas_global.vi" "Pre Setup String"() -> (w902:string)
          n440 = call "Get_Characters_from_string.vi"("Input string"=w902, "Variable name"="Skip_Block_Numbers_(eg 1;2;5;12)") -> ("Status"=w900:enum16{"Char in string", "Char not in string"}, "Value"=w899:string)  [unwired: 1 in]
          n441 = case shown="\"Char in string\"" w900 {
            tunnel: w899 -> [w906 _]
            tunnel: [w904 i32[] []] -> w898
            frame "Char in string" {
              n442 = call "Get_array_values_fr_String.vi"("String Value"=w906) -> ("Numeric Array"=w905:dbl[])  [unwired: 1 out]
              n443 = To Long Integer(number=w905) -> (32bit integer=w904:i32[])
            }
            frame "Char not in string" {
            }
          }
          n444 = global write "Meas_global.vi" "Blocks to Skip"(w898) -> ()
        }
      }
    }
    frame #8 {
      n445 = global read "Meas_global.vi" "Pre Setup String"() -> (w910:string)
      n446 = for {
        tunnel: [w921] -> w913 mode=indexing
        tunnel: w912 -> [w918] mode=indexing
        tunnel: w911 -> [w920] mode=indexing
        tunnel: w910 -> [w919]
        n447 = Unbundle By Name(w918) -> ("Code name"=w917:string)
        n448 = Concatenate Strings(w917, "_Av_SamplingRate" ("string")) -> (w915:string)
        n449 = call "Get_value_from_string.vi"("Input string"=w919, "Variable name"=w915) -> ("Value"=w914:dbl)  [unwired: 1 in, 1 out]
        n450 = Bundle By Name(cluster=w918, "Calib File"=w920, "Av Sampling Rate"=w914) -> (w921:T8)
      }
      "Analysis Info cluster" <- w913
    }
  }
